vi "Read Response.vi"(8 "error in (no error)":errorcluster, 10 "Commands":T1, 11 "Force Test Stand in":refnum<class "Force Test Stand.lvclass">) -> (0 "error out":errorcluster, 3 "Force Test Stand out":refnum<class "Force Test Stand.lvclass">)   [LabVIEW 2018, in "Force Test Stand.lvlib" / "Force Test Stand.lvclass"]
uses:
  Force Test Stand.lvclass
  Custom Controls/Commands.ctl
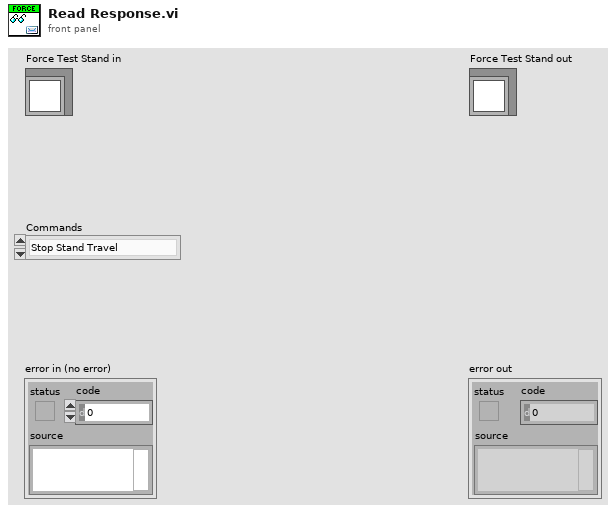
[diagram p1: front panel]
types:
  T1 = typedef "Force Test Stand.lvlib/Force Test Stand.lvclass/Commands.ctl" = enum16{"Stop Stand Travel", "Start Travel Down (Left)", "Start Travel Up (Right)", "Get Travel Upper Limit", "Get Travel Lower Limit", "Set Travel Upper Limit", "Set Travel Lower Limit", "Get Travel Value", "Set Travel Units (mm)", "Set Travel Units (in)", "Reset Travel to Zero", "Get Speed ", "Set Speed", "Set Speed to Min", "Set Speed to Max", "Get Force Value", "Get Force Units", "Set Force Units (lbF)", "Get Stand Status", "Set Cycle Mode", "Set Limit Mode", "Set Manual Mode", "Set No. Cycles", "Get Travel/Force Values", "Get Completed Cycles", "Get Cycles Setpoint", "Reset Cycles Counter", "Zero Force Gauge", "Set Force Upper Limit", "Set Force Lower Limit", "Get Travel Units", "Get Speed Units", "Default", "Set Force Units (N)", "Set Force Units (kgF)", "Set Force Units (ozF)", "Set Force Units (gF)", "Set Force Real Time Mode", "Set Force Peak Tension Mode", "Set Force Peak Compression Mode", "Set Force High Set-Point", "Set Force Low Set-Point", "Gauge Transmit with Units", "Gauge Transmit w/o Units", "Get Peak Compression Force", "Get Peak Tension Force", "Get Real Time Force", "Disable Force High Limit", "Disable Force Low Limit", "Send Speed Setting to Stand"}
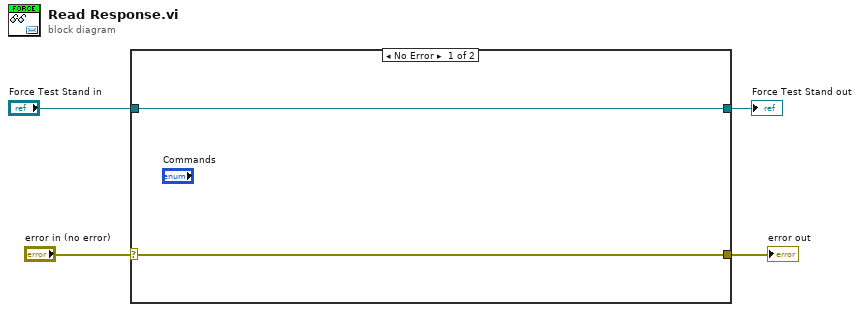
[diagram p0: block diagram]
diagram:
  n1 = case shown="No Error" "error in (no error)" {
    selector: "error in (no error)" -> [w5 w8]
    tunnel: [w5 w8] -> w3
    tunnel: [w6 w7] -> w1
    tunnel: "Force Test Stand in" -> [w6 w7]
    frame No Error {
    }
    frame Error {
    }
  }
  "error out" <- w3
  "Force Test Stand out" <- w1
